vi "Write ASCII or Unicode.vi"(0 "PDF Report IN":refnum<class "PDF Report Class.lvclass">, 7 "ASCII or Unicode":T1={"Type"=enum."ASCII", "Direction"=enum."Default"}, 11 "error in (no error)":errorcluster) -> (4 "PDF Report OUT":refnum<class "PDF Report Class.lvclass">, 15 "error out":errorcluster)   [LabVIEW 2019]
doc: "Version 2.0\nDeveloped by Jean-Marc Simard\nCopyright © 2012, Exaprom Inc.\nAll rights reserved.\nLicense: BSD\n\nWith iTextSharp 4.1.6 (http://itextsharp.sourceforge.net)\nunder Mozilla Public License Version 1.1\n(http://www.mozilla.org/MPL/MPL-1.1.html)"
uses:
  <userlib>/Exaprom PDF/LV Class/PDF Report Class/PDF Report Class.lvclass
  <userlib>/Exaprom PDF/Controls/Text Controls/Unicode/Character type with Select.ctl
  <userlib>/Exaprom PDF/Controls/Text Controls/Unicode/Writing direction with Select.ctl
  <userlib>/Exaprom PDF/LV Class/Fonts Class/Font Class.lvclass
  <userlib>/Exaprom PDF/Controls/Text Controls/Unicode/ASCII or Unicode with Select.ctl
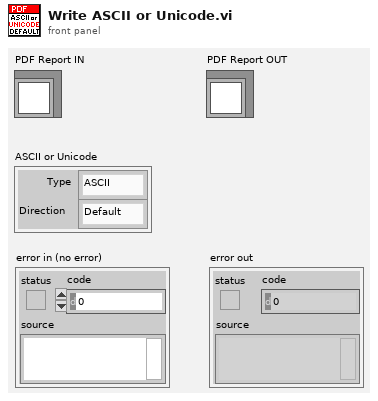
[diagram p1: front panel]
types:
  T1 = typedef "ASCII or Unicode with Select.ctl" = cluster{"Type":T2, "Direction":T3}
  T2 = typedef "Character type with Select.ctl" = enum16{"Select", "ASCII", "Unicode"}
  T3 = typedef "Writing direction with Select.ctl" = enum16{"Select", "Default", "NO BIDI", "LTR", "RTL"}
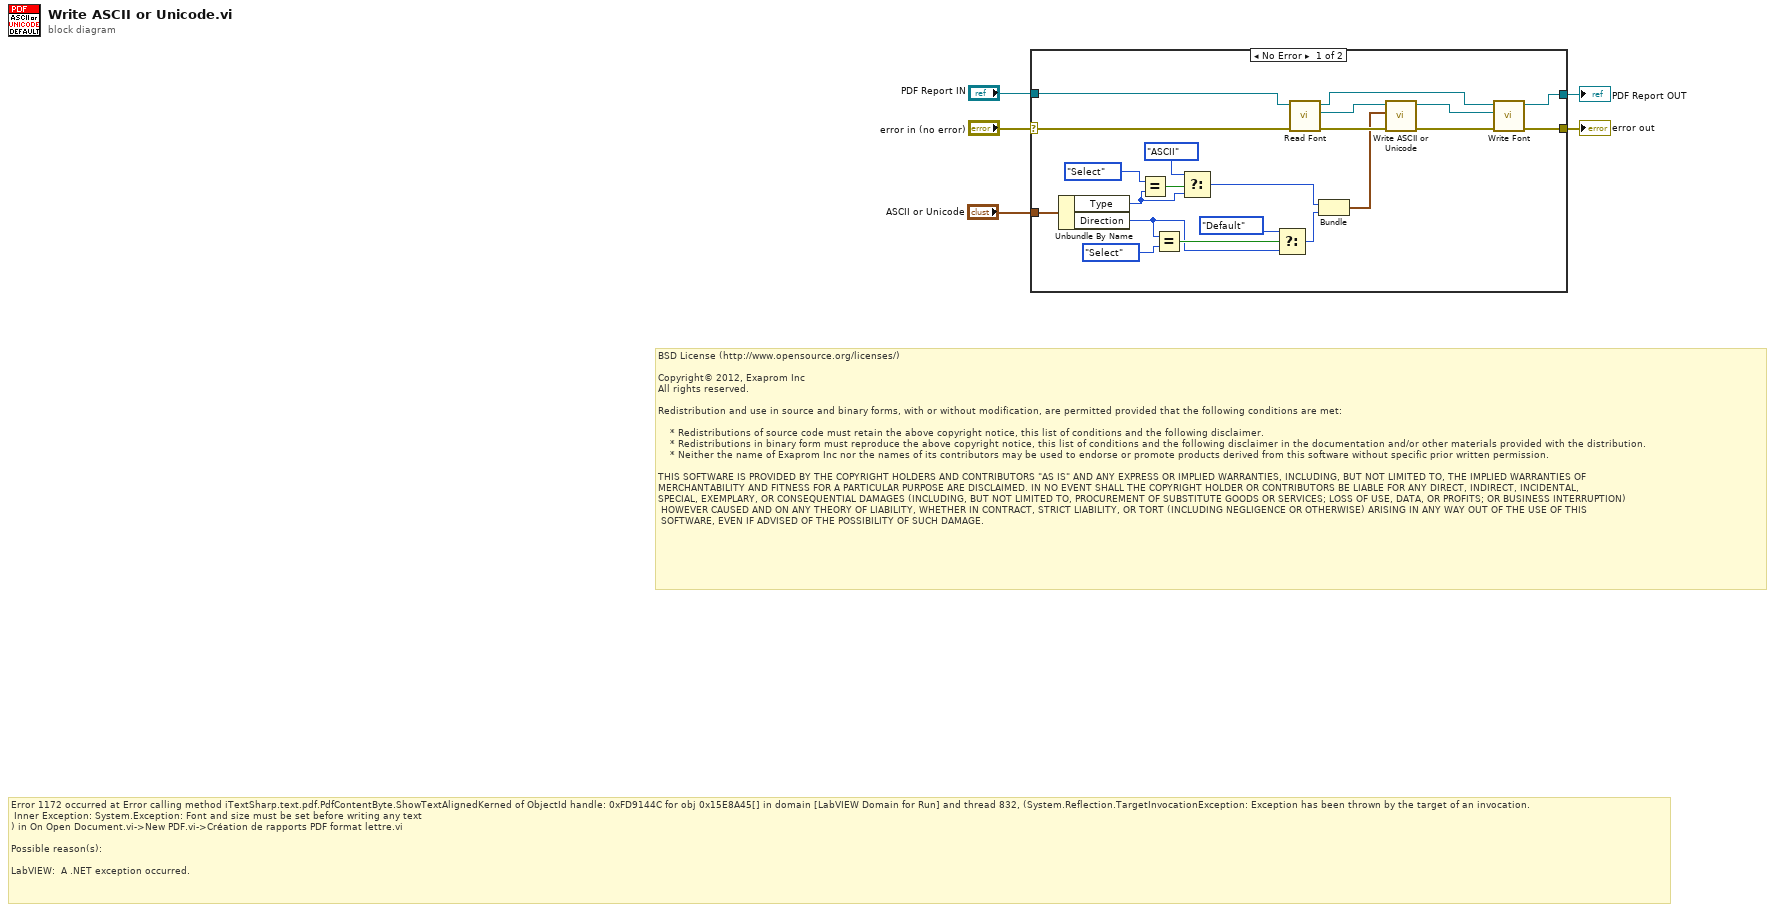
[diagram p0: block diagram]
diagram:
  # "Error 1172 occurred at Error calling method iTextSharp.text.pdf.PdfContentByte.ShowTextAlignedKerned of ObjectId handle: 0xFD9144C for obj 0x15E8A45[] in domain [LabVIEW Domain for Run] and thread 832, (System.Reflection.TargetInvocationException: Exception has been thrown by the target of an invocation.\n\tInner Exception: System.Exception: Font and size must be set before writing any text\n) in On Open Document.vi->New PDF.vi->Création de rapports PDF format lettre.vi\n\nPossible reason(s):\n\nLabVIEW:  A .NET exception occurred."
  # "BSD License (http://www.opensource.org/licenses/)\n\nCopyright© 2012, Exaprom Inc\nAll rights reserved.\n\nRedistribution and use in source and binary forms, with or without modification, are permitted provided that the following conditions are met:\n\n    * Redistributions of source code must retain the above copyright notice, this list of conditions and the following disclaimer.\n    * Redistributions in binary form must reproduce the above copyright notice, this list of conditions and the following disclaimer in the documentation and/or other materials provided with the distribution.\n    * Neither the name of Exaprom Inc nor the names of its contributors may be used to endorse or promote products derived from this software without specific prior written permission.\n\nTHIS SOFTWARE IS PROVIDED BY THE COPYRIGHT HOLDERS AND CONTRIBUTORS \"AS IS\" AND ANY EXPRESS OR IMPLIED WARRANTIES, INCLUDING, BUT NOT LIMITED TO, THE IMPLIED WARRANTIES OF \nMERCHANTABILITY AND FITNESS FOR A PARTICULAR PURPOSE ARE DISCLAIMED. IN NO EVENT SHALL THE COPYRIGHT HOLDER OR CONTRIBUTORS BE LIABLE FOR ANY DIRECT, INDIRECT, INCIDENTAL,\nSPECIAL, EXEMPLARY, OR CONSEQUENTIAL DAMAGES (INCLUDING, BUT NOT LIMITED TO, PROCUREMENT OF SUBSTITUTE GOODS OR SERVICES; LOSS OF USE, DATA, OR PROFITS; OR BUSINESS INTERRUPTION)\n HOWEVER CAUSED AND ON ANY THEORY OF LIABILITY, WHETHER IN CONTRACT, STRICT LIABILITY, OR TORT (INCLUDING NEGLIGENCE OR OTHERWISE) ARISING IN ANY WAY OUT OF THE USE OF THIS\n SOFTWARE, EVEN IF ADVISED OF THE POSSIBILITY OF SUCH DAMAGE."
  n1 = case shown="No Error" "error in (no error)" {
    selector: "error in (no error)" -> [w24 w28]
    tunnel: "PDF Report IN" -> [w23 w27]
    tunnel: [w18 w27] -> w4
    tunnel: [w21 w28] -> w3
    tunnel: "ASCII or Unicode" -> [w17 _]
    frame No Error {
      n2 = Unbundle By Name(w17) -> ("Type"=w13:T2, "Direction"=w10:T3)
      n3 = Equal?(x=Character_type_with_Select."Select" ("Type"), y=w13) -> (x = y?=w15:bool)
      n4 = Equal?(x=w10, y=Writing_direction_with_Select."Select" ("Direction")) -> (x = y?=w11:bool)
      n5 = Select(t=Character_type_with_Select."ASCII" ("Type"), s=w15, f=w13) -> (s? t:f=w8:T2)
      n6 = Select(t=Writing_direction_with_Select."Default" ("Direction"), s=w11, f=w10) -> (s? t:f=w7:T3)
      n7 = call-dynamic "Read Font.vi"("error in (no error)"=w24, "PDF Report Class in"=w23) -> ("error out"=w25:errorcluster, "Font Class.lvclass"=w26:refnum<class "Font Class.lvclass">, "PDF Report Class out"=w19:refnum<class "PDF Report Class.lvclass">)  [unwired: 7 in]
      n8 = Bundle("Type"=w8, "Direction"=w7) -> (w6:cluster{"Type":T2, "Direction":T3})  [unwired: 1 in]
      n9 = call-dynamic "Write ASCII or Unicode.vi"("error in (no error)"=w25, "ASCII or Unicode"=w6, "Font Class in"=w26) -> ("error out"=w22:errorcluster, "Font Class out"=w20:refnum<class "Font Class.lvclass">)  [unwired: 7 in]
      n10 = call-dynamic "Write Font.vi"("error in (no error)"=w22, "Font Class.lvclass"=w20, "PDF Report Class in"=w19) -> ("error out"=w21:errorcluster, "PDF Report Class out"=w18:refnum<class "PDF Report Class.lvclass">)  [unwired: 7 in]
    }
    frame Error {
    }
  }
  "PDF Report OUT" <- w4
  "error out" <- w3
